vi "LU_TableMap_Read.vi"(8 "error in (no error)":errorcluster, 10 "TableName":string, 11 "KDBConnection in":refnum<class "DBC.lvclass">) -> (0 "error out":errorcluster, 1 "TableType":T1, 2 "TableName Out":string, 3 "KDBConnection out":refnum<class "DBC.lvclass">)   [LabVIEW 2020, in "ORM_DBC_Kdb.lvlib" / "DBC.lvclass"]
uses:
  DBC.lvclass
  kdb_TableType_enum.ctl
  DBC.lvclass/DBC.ctl
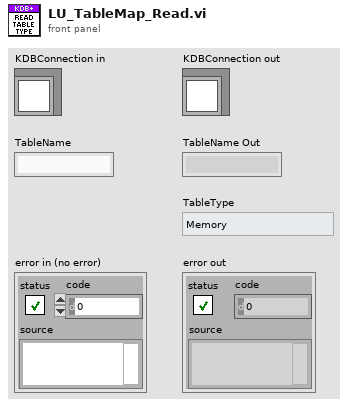
[diagram p1: front panel]
types:
  T1 = typedef "ORM_DBC_Kdb.lvlib/DBC.lvclass/kdb_TableType_enum.ctl" = enum16{"Memory", "Disk_Serialized", "Disk_Splayed", "Disk_Partitioned", "Other"}
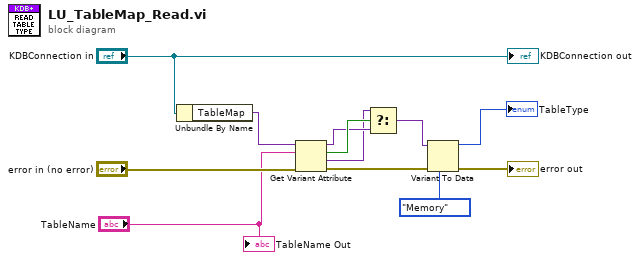
[diagram p0: block diagram]
diagram:
  n1 = Unbundle By Name("KDBConnection in") -> ("TableMap"=w11:variant)
  n2 = Get Variant Attribute(Variant=w11, name="TableName", error in="error in (no error)") -> (duplicate Variant=w7:variant, found=w8:bool, value=w6:variant, error out=w5:errorcluster)  [unwired: 1 in]
  n3 = Select(t=w6, s=w8, f=w7) -> (s? t:f=w3:variant)
  n4 = Variant To Data(error in=w5, type=kdb_TableType_enum."Memory" ("TableType"), Variant=w3) -> (data=→"TableType":T1, error out=→"error out":errorcluster)
  "KDBConnection out" <- "KDBConnection in"
  "TableName Out" <- "TableName"
